vi "Process.vi"(8 "error in":errorcluster, 11 "Plugin in":refnum<class "Statistic.lvclass">) -> (0 "error out":errorcluster, 3 "Plugin out":refnum<class "Statistic.lvclass">)   [LabVIEW 2025, in "Statistic.lvlib" / "Statistic.lvclass"]
uses:
  Statistic.lvclass
  C:/Program Files/National Instruments/LabVIEW 2025/vi.lib/FlexLogger/SDK/PluginSDK.lvlibp/PEFClasses/SDK/Plugin/Plugin.lvclass
  Statistic.lvclass/Statistic.ctl
  <vilib>/FlexLogger/SDK/PluginSDK.lvlibp/PEFClasses/SDK/Plugin/DataHelpers/Write 1D Wfm (DBL)_v2.vi
  C:/Program Files/National Instruments/LabVIEW 2025/vi.lib/FlexLogger/SDK/PluginSDK.lvlibp/PEFClasses/SDK/Processing Element/Processing Element.lvclass
  C:/Users/Tester/Documents/LabVIEW Projects/FlexLogger IO Plug-ins/Statistic/Statistic.lvclass
  <vilib>/FlexLogger/SDK/PluginSDK.lvlibp/PEFClasses/SDK/Plugin/Plugin.lvclass
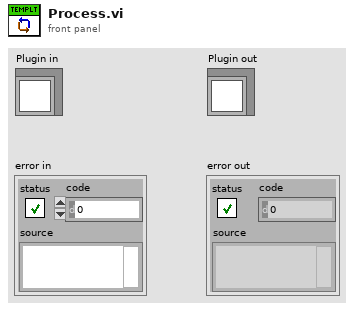
[diagram p1: front panel]
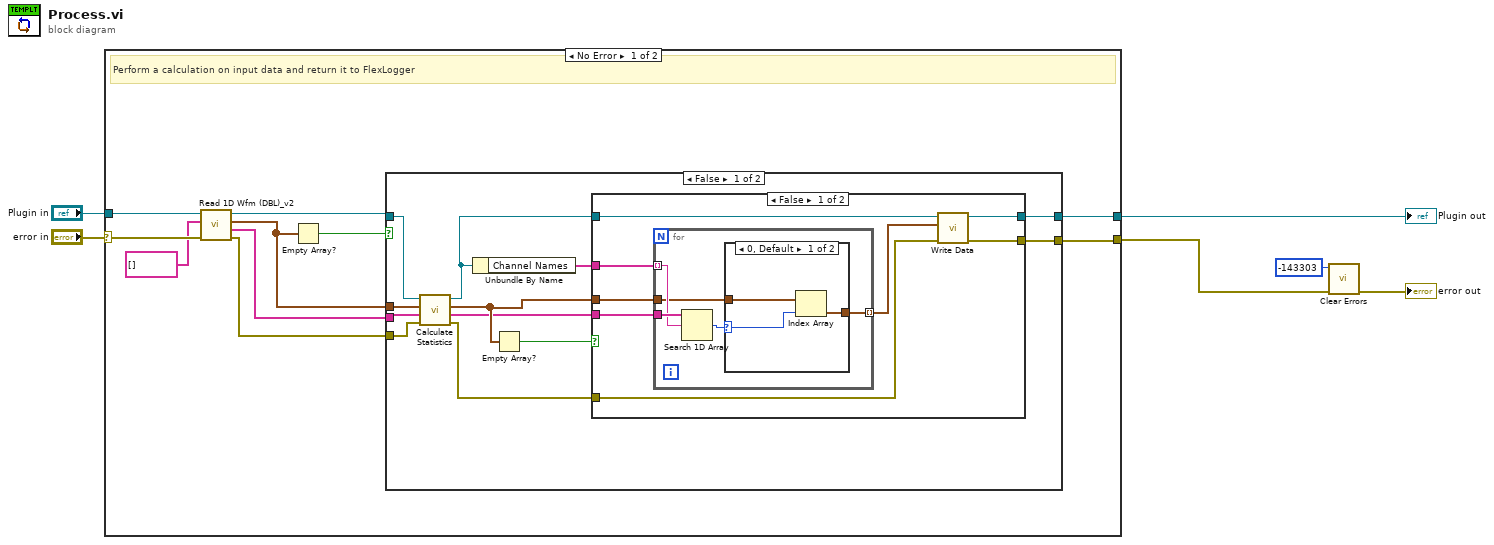
[diagram p0: block diagram]
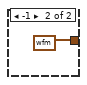
[diagram p2: hidden frame]
diagram:
  n1 = case shown="No Error" "error in" {
    selector: "error in" -> [w15 w50]
    tunnel: [w8 w51] -> w3
    tunnel: "Plugin in" -> [w16 w51]
    tunnel: [w7 w50] -> w2
    frame No Error {
      # "Perform a calculation on input data and return it to FlexLogger"
      n2 = call <vilib>:"Read 1D Wfm (DBL)_v2.vi"("error in (no error)"=w15, "Unique Identifiers (empty = all)"=string[] [] ("Unique Channel Identifers (empty = all)"), "Plugin in"=w16) -> ("error out"=w9:errorcluster, "Stream Names"=w10:string[], "Data"=w11:waveform(dbl)[], "Plugin out"=w12:refnum<class "Statistic.lvclass">)  [unwired: 5 in]
      n3 = Empty Array?(array=w11) -> (empty?=w13:bool)
      n4 = case shown="False" w13 {
        tunnel: w12 -> [w25 w49]
        tunnel: [w28 w49] -> w8
        tunnel: w9 -> [w21 w48]
        tunnel: w11 -> [w23 _]
        tunnel: w10 -> [w22 _]
        tunnel: [w17 w48] -> w7
        frame False {
          n5 = call-dynamic "Calculate Statistics.vi"("error in (no error)"=w21, "Stream Names"=w22, "Data"=w23, "Statistic in"=w25) -> ("error out"=w18:errorcluster, "Statistic Channels"=w19:string[], "Statistic Waveforms"=w20:waveform(dbl)[], "Statistic out"=w24:refnum<class "Statistic.lvclass">)  [unwired: 4 in]
          n6 = Unbundle By Name(w24) -> ("Channel Names"=w27:string[])
          n7 = Empty Array?(array=w20) -> (empty?=w26:bool)
          n8 = case shown="False" w26 {
            tunnel: [w36 w47] -> w28
            tunnel: w27 -> [w35 _]
            tunnel: w19 -> [w30 _]
            tunnel: w24 -> [w34 w47]
            tunnel: w20 -> [w32 _]
            tunnel: w18 -> [w31 w46]
            tunnel: [w29 w46] -> w17
            frame False {
              n9 = for {
                tunnel: w35 -> [w40] mode=indexing
                tunnel: w32 -> [w39]
                tunnel: w30 -> [w41]
                tunnel: [w37] -> w33 mode=indexing
                n10 = Search 1D Array(1D array=w41, element=w40) -> (index of element=w38:i32)  [unwired: 1 in]
                n11 = case shown="0, Default" w38 {
                  selector: w38 -> [w43 _]
                  tunnel: w39 -> [w44 _]
                  tunnel: [w42 waveform(dbl) {"t0"=timestamp(0 s since 1904-01-01), "dt"=1.0, "Y"=[]} ("Waveform")] -> w37
                  frame 0, Default {
                    n12 = Index Array(array=w44, index=w43) -> (element=w42:waveform(dbl))
                  }
                  frame -1 {
                  }
                }
              }
              n13 = call-poly <vilib>:"Write Data.vi"("error in (no error)"=w31, "Data"=w33, "Plugin in"=w34) -> ("error out"=w29:errorcluster, "Plugin out"=w36:refnum<class "Statistic.lvclass">)  [unwired: 7 in]
            }
            frame True {
            }
          }
        }
        frame True {
        }
      }
    }
    frame Error {
    }
  }
  "Plugin out" <- w3
  n14 = call <vilib>:"Clear Errors.vi"("error in (no error)"=w2, "specific error code to clear (0: all)"=-143303) -> ("error out"=→"error out":errorcluster)  [unwired: 4 in, 1 out]
